vi "5-6_Fan Control with Long Push Stop(LatchWhenReleased).vi"() -> ()   [LabVIEW 2014]
doc: "This example demonstrates how to read one channel of digital input from a LINX device.\n------------------------------------\nAuther: Koji Ohashi\nChanged: Hirotake Watashima\nCopyright (c) 2020 Japan LabVIEW Users Group, Volunteer members.\nThis VI is released under the MIT License.\nhttp://opensource.org/licenses/mit-license.php\n------------------------------------"
uses:
  <vilib>/MakerHub/LINX/LMH-LINX.lvlib
  <vilib>/MakerHub/LINX/Public/Utilities/Open Serial.vi
  <vilib>/MakerHub/LINX/Public/Peripherals/Digital/Digital Read 1 Chan.vi
  <vilib>/MakerHub/LINX/Public/Peripherals/PWM/PWM Set Duty Cycle 1 Chan.vi
panel:
  in  "Serial Port":refnum<visa-resource-name>
  out "Duty Cycle":dbl
  in  "PWM Channel":u8=9
  out "Count":u32
  out "DI Value":bool
  in  "DI Channel":u8=8
  in  "Stop Button":bool
  # "LINX Device Settings"
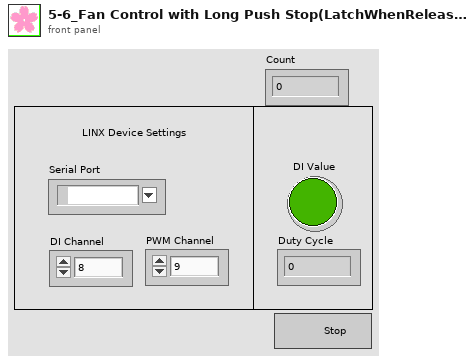
[diagram p1: front panel]
types:
  T1 = typedef "LMH-LINX.lvlib/LINX Ref.ctl" = cluster{"IO":T2, "Interface":T3, "LINX Device Config":T4}
  T2 = typedef "LMH-LINX.lvlib/Platform.ctl" = enum16{"Remote", "Local"}
  T3 = typedef "LMH-LINX.lvlib/Interface.ctl" = enum16{"Serial", "TCP"}
  T4 = typedef "LMH-LINX.lvlib/Device.lvlib/LINX Device Config.ctl" = cluster{"Interface":T3, "COM Port":refnum<visa-resource-name>, "TCP Configuration":T5, "Device Family":u8, "Device ID":u8, "Device Name":string, "TCP Ref":refnum<k5>, "Channels":T6}
  T5 = typedef "LMH-LINX.lvlib/Device.lvlib/TCP Config.ctl" = cluster{"IP Address":string, "Port":u16}
  T6 = typedef "LMH-LINX.lvlib/Channels.ctl" = cluster{"DI":u8[], "DO":u8[], "AI":u8[], "AO":u8[], "PWM":u8[], "QE":u8[], "UART":u8[], "I2C 2":u8[], "SPI":u8[], "CAN":u8[], "Servo":u8[], "AI Ref (V)":dbl, "AI Resolution (Bits)":u8, "AO Ref (V)":dbl, "AO Resolution (Bits)":u8}
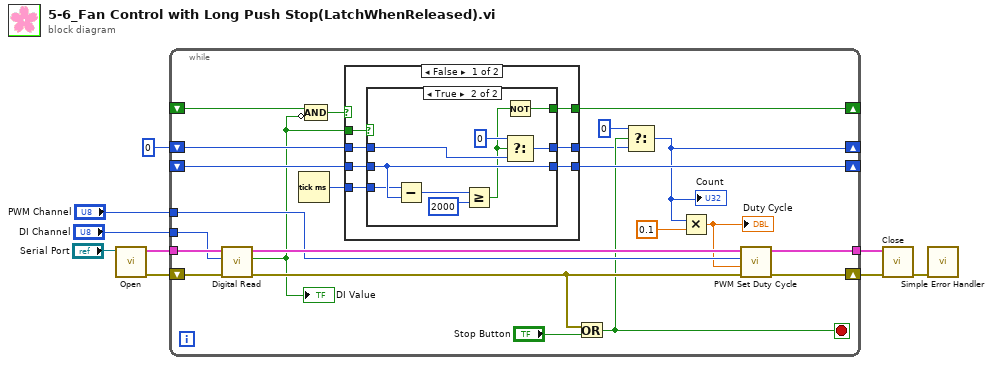
[diagram p0: block diagram]
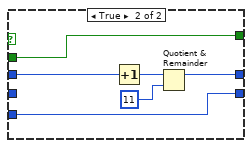
[diagram p3: hidden frame]
diagram:
  n1 = call-poly <vilib>:"Open.vi"("Serial Port"="Serial Port") -> ("Error Out"=w8:errorcluster, "LINX Resource"=w9:T1)  [unwired: 8 in, 1 out]
  n2 = while {
    tunnel: w9 -> [w31]
    tunnel: [w24] -> w7
    shift-right: [w23] -> w6
    shift-left: w8 -> [w30]
    tunnel: "DI Channel" -> [w29]
    shift-right: [w11] -> _
    shift-left: _ -> [w28]
    shift-right: [w10] -> _
    shift-left: u32 0 -> [w26]
    tunnel: "PWM Channel" -> [w21]
    shift-right: [w20] -> _
    shift-left: _ -> [w19]
    stop <- w15 stop-if-true
    n3 = call-poly <vilib>:"Digital Read.vi"("Error In"=w30, "DI Channel"=w29, "LINX Resource"=w31) -> ("Error Out"=w16:errorcluster, "DI Value"=w12:bool, "LINX Resource"=w25:T1)  [unwired: 6 in]
    "DI Value" <- w12
    n4 = Tick Count (ms)() -> (millisecond timer value=w18:u32)
    n5 = Compound Arithmetic op=AND ("複合演算")(w28, invert w12) -> (w27:bool)
    n6 = case shown="FALSE" w27 {
      tunnel: w26 -> [w35 w56]
      tunnel: [w34 w54] -> w14
      tunnel: w12 -> [w39 w52]
      tunnel: [w36 w53] -> w20
      tunnel: w19 -> [w38 _]
      tunnel: w18 -> [w37 w53]
      tunnel: [w33 w52] -> w11
      frame False {
        n7 = case shown="TRUE" w39 {
          selector: w39 -> [w40 _]
          tunnel: [w42 w51] -> w36
          tunnel: w38 -> [_ w51]
          tunnel: w37 -> [w42 w50]
          tunnel: w35 -> [w41 w47]
          tunnel: [w41 w46] -> w34
          tunnel: [w40 w43] -> w33
          frame False {
          }
          frame True {
            n8 = Subtract(x=w50, y=w51) -> (x-y=w49:u32)
            n9 = Greater Or Equal?(x=w49, y=u32 2000) -> (x >= y?=w44:bool)
            n10 = Not(x=w44) -> (.not. x?=w43:bool)
            n11 = Select(t=u32 0, s=w44, f=w47) -> (s? t:f=w46:u32)
          }
        }
      }
      frame True {
        n12 = Increment(x=w56) -> (x+1=w55:u32)
        n13 = Quotient & Remainder(x=w55, y=u32 11) -> (x-y*floor(x/y)=w54:u32)  [unwired: 1 out]
      }
    }
    n14 = Or(x=w16, y="Stop Button") -> (x .or. y?=w15:bool)
    n15 = Select(t=u32 0, s=w15, f=w14) -> (s? t:f=w10:u32)
    "Count" <- w10
    n16 = Multiply(x=w10, y=0.1) -> (x*y=w17:dbl)
    "Duty Cycle" <- w17
    n17 = call-poly <vilib>:"PWM Set Duty Cycle.vi"("Error In"=w16, "Duty Cycle (0-1)"=w17, "PWM Channel"=w21, "LINX Resource"=w25) -> ("Error Out"=w23:errorcluster, "LINX Resource"=w24:T1)  [unwired: 6 in]
  }
  n18 = call <vilib>:"Close.vi"("Error In"=w6, "LINX Resource"=w7) -> ("Error Out"=w5:errorcluster)  [unwired: 9 in]
  n19 = call <vilib>:"Simple Error Handler.vi"("error in (no error)"=w5) -> ()  [unwired: 4 in, 5 out]
